vi "wait_init_02.vi"   [LabVIEW 2011]
uses:
  wait_globals.vi
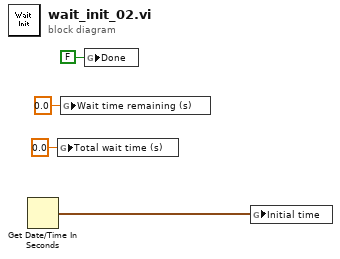
[diagram p0: block diagram]
diagram:
  n1 = Get Date/Time In Seconds() -> (seconds since 1Jan1904=w1:timestamp)
  n2 = global write "wait_globals.vi" "Total wait time (s)"(0.0 ("Total wait time (s)")) -> ()
  n3 = global write "wait_globals.vi" "Wait time remaining (s)"(0.0 ("Wait time remaining (s)")) -> ()
  n4 = global write "wait_globals.vi" "Done"(FALSE ("Done")) -> ()
  n5 = global write "wait_globals.vi" "Initial time"(w1) -> ()
